vi "Drive Button Pressed Handler.vi"(10 "Button X":bool, 11 "Button B":bool) -> (2 "Button X Pressed":bool, 3 "Button B Pressed":bool)   [LabVIEW 2019]
uses:
  afdaa0f5-9f49-4630-b5f7-78f3a1fe44a9.vi
  24f32ee9-c2f2-443f-ad5d-076de7e5996f.vi
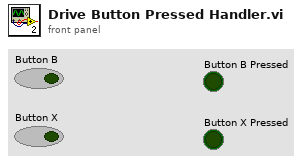
[diagram p1: front panel]
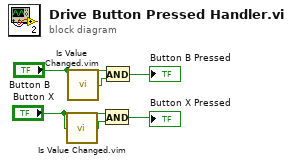
[diagram p0: block diagram]
diagram:
  n1 = call "Is Value Changed.vim"("value"="Button X") -> ("changed or first call?"=w4:bool)
  n2 = call "Is Value Changed.vim"("value"="Button B") -> ("changed or first call?"=w5:bool)
  n3 = And(x="Button X", y=w4) -> (x .and. y?=→"Button X Pressed":bool)
  n4 = And(x="Button B", y=w5) -> (x .and. y?=→"Button B Pressed":bool)
